vi "Create Hidden Files.vi"(9 "TemplatePath":path, 11 "DataFilePath":path) -> (1 "Specs Path":path, 2 "Stats path":path, 3 "Data Path":path)   [LabVIEW 2013]
panel:
  out "error out":errorcluster
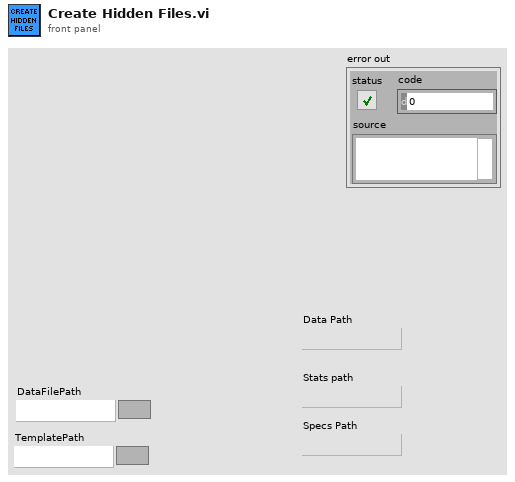
[diagram p1: front panel]
types:
  T1 = enum16{"open", "replace", "create", "open or create", "replace or create", "replace or create with confirmation"}
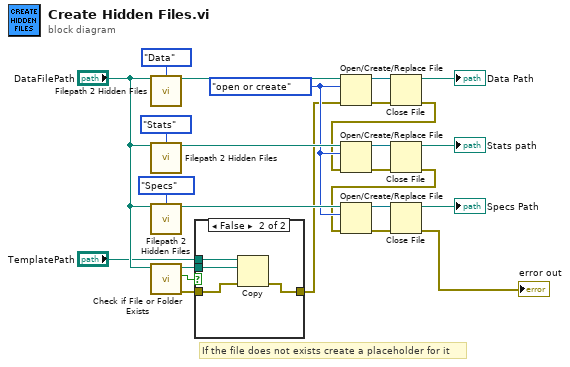
[diagram p0: block diagram]
diagram:
  w19 = T1."open or create" ("operation (0:open)")
  # "If the file does not exists create a placeholder for it"
  n1 = call "Filepath 2 Hidden Files.vi"("DataFilePath"="DataFilePath", "Enum"=enum16{"Data", "Stats", "Specs"}."Data") -> ("HiddenFilePath"=w20:path)  [unwired: 13 in]
  n2 = call "Filepath 2 Hidden Files.vi"("DataFilePath"="DataFilePath", "Enum"=enum16{"Data", "Stats", "Specs"}."Stats") -> ("HiddenFilePath"=w21:path)  [unwired: 13 in]
  n3 = call "Filepath 2 Hidden Files.vi"("DataFilePath"="DataFilePath", "Enum"=enum16{"Data", "Stats", "Specs"}."Specs") -> ("HiddenFilePath"=w22:path)  [unwired: 13 in]
  n4 = call <vilib>:"Check if File or Folder Exists.vi"("path"="DataFilePath") -> ("error out"=w4:errorcluster, "file or folder exists?"=w6:bool, "dup path"=w5:path)  [unwired: 8 in]
  n5 = case shown="False" w6 {
    tunnel: w5 -> [_ w30]
    tunnel: w4 -> [w26 w28]
    tunnel: "TemplatePath" -> [_ w29]
    tunnel: [w26 w27] -> w2
    frame True {
    }
    frame False {
      n6 = Copy(8:w28, 10:w30, 11:w29) -> (0:w27:errorcluster)  [unwired: 2 in, 2 out]
    }
  }
  n7 = Open/Create/Replace File(file path (use dialog)=w20, error in=w2, operation (0:open)=w19) -> (refnum out=w14:refnum<file>, error out=w18:errorcluster)  [unwired: 3 in, 1 out]
  n8 = Close File(refnum=w14, error in=w18) -> (path=→"Data Path":path, error out=w12:errorcluster)
  n9 = Open/Create/Replace File(file path (use dialog)=w21, error in=w12, operation (0:open)=w19) -> (refnum out=w15:refnum<file>, error out=w16:errorcluster)  [unwired: 3 in, 1 out]
  n10 = Close File(refnum=w15, error in=w16) -> (path=→"Stats path":path, error out=w11:errorcluster)
  n11 = Open/Create/Replace File(file path (use dialog)=w22, error in=w11, operation (0:open)=w19) -> (refnum out=w13:refnum<file>, error out=w17:errorcluster)  [unwired: 3 in, 1 out]
  n12 = Close File(refnum=w13, error in=w17) -> (path=→"Specs Path":path, error out=→"error out":errorcluster)
